vi "GetStatus.vi"(8 "error in":errorcluster, 11 "VISA resource name":refnum<visa-resource-name>) -> (0 "error out":errorcluster, 1 "Status word":i32, 2 "Status string":string, 3 "VISA resource name out":refnum<visa-resource-name>)   [LabVIEW 2023, in "Thermotron 8800.lvlib"]
doc: "STAT\nCommand name: Send status word\nCommand type: System status\nDescription: The 8800 returns one byte of coded-decimal data to indicate the status of the 8800. The byte is defined below:\n1 Run program\n2 Hold program\n4 Suspend program\n8 Undefined\n16 Run manual\n32 Hold manual\n64 Undefined\n128 Undefined\nSyntax: STAT?\nData type: Coded decimal\nQuery example: STAT?\n8800 response: 16 (The 8800 is in run manual mode.)"
uses:
  Thermotron 8800.lvlib
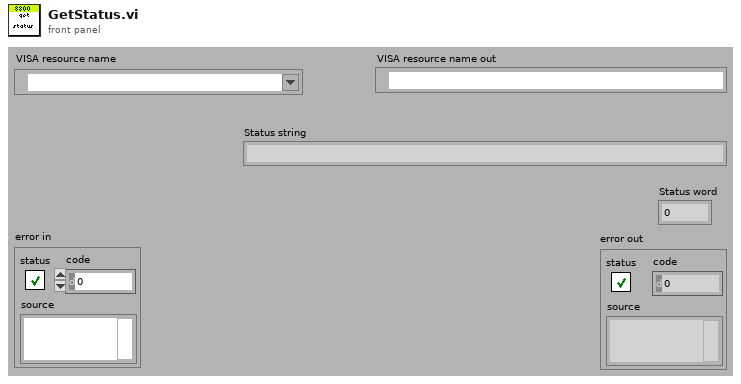
[diagram p1: front panel]
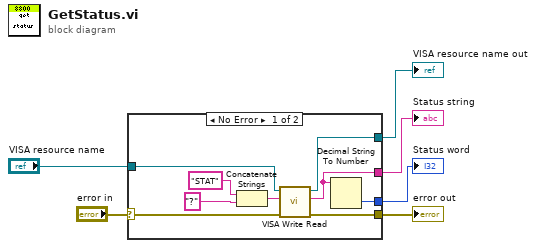
[diagram p0: block diagram]
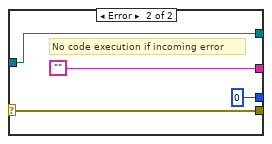
[diagram p2: hidden frame]
diagram:
  n1 = case shown="No Error" "error in" {
    selector: "error in" -> [w13 w19]
    tunnel: [w12 w19] -> w5
    tunnel: "VISA resource name" -> [w11 w16]
    tunnel: [w10 w16] -> w3
    tunnel: [w9 ""] -> w2
    tunnel: [w8 0] -> w1
    frame No Error {
      n2 = Concatenate Strings("STAT" ("8800 Command"), "?" ("8800 Command")) -> (w15:string)
      n3 = call "VISA Write Read.vi"("error in (no error)"=w13, "8800 Command"=w15, "VISA Refnum in"=w11) -> ("error out"=w12:errorcluster, "read buffer"=w9:string, "VISA Refnum out"=w10:refnum<visa-resource-name>)  [unwired: 6 in]
      n4 = Decimal String To Number(string=w9) -> (number=w8:i32)  [unwired: 2 in, 1 out]
    }
    frame Error {
      # "No code execution if incoming error"
    }
  }
  "error out" <- w5
  "VISA resource name out" <- w3
  "Status string" <- w2
  "Status word" <- w1
